vi "Logistic CDF.vi"(9 "b":dbl=1.0, 10 "a":dbl=1.0, 11 "x":dbl) -> (0 "error":i32, 3 "cdf(x)":dbl=0.2689414213699951)   [LabVIEW 2017, in "NI_Gmath.lvlib"]
doc: "Computes the continuous cumulative distribution function (CDF), or the probability that the random variate X, where X describes the selected distribution type, has a value less than or equal to <B>x</B>. You must manually select the polymorphic instance to use."
uses:
  <vilib>/gmath/NI_Gmath.lvlib
  <vilib>/gmath/statdist.llb/st_error_code.ctl
panel:
  # "Logistic CDF"
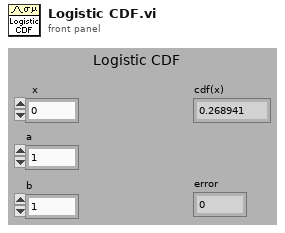
[diagram p1: front panel]
types:
  T1 = typedef "NI_Gmath.lvlib/st_error_code.ctl" = i32
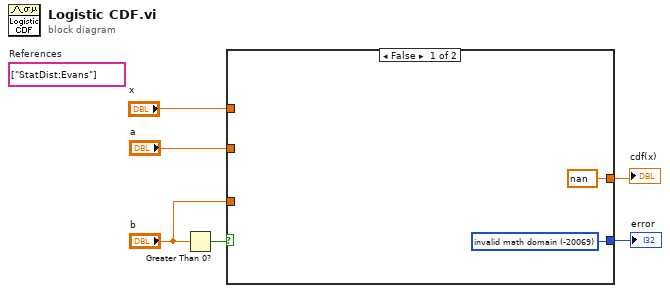
[diagram p0: block diagram]
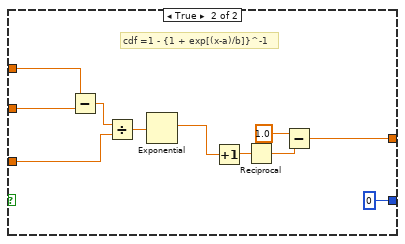
[diagram p2: hidden frame]
diagram:
  (unwired) string[] ["StatDist:Evans"]  # References
  n1 = Greater Than 0?(x="b") -> (x > 0?=w1:bool)
  n2 = case shown="False" w1 {
    tunnel: "b" -> [_ w14]
    tunnel: [w7 0 ("invalid math domain")] -> w2
    tunnel: [nan w9] -> w3
    tunnel: "x" -> [_ w18]
    tunnel: "a" -> [_ w17]
    frame False {
      w7 = T1 -20069 items=["invalid math domain"=-20069, "Fourier interpolation size m >= n"=-20070, "empty array"=-20003] ("stat interp error code")
    }
    frame True {
      # "cdf =1 - {1 + exp[(x-a)/b]}^-1"
      n3 = Subtract(x=w18, y=w17) -> (x-y=w16:dbl)
      n4 = Divide(x=w16, y=w14) -> (x/y=w15:dbl)
      n5 = Exponential(1:w15) -> (0:w13:dbl)
      n6 = Increment(x=w13) -> (x+1=w11:dbl)
      n7 = Reciprocal(x=w11) -> (1/x=w10:dbl)
      n8 = Subtract(x=1.0, y=w10) -> (x-y=w9:dbl)
    }
  }
  "cdf(x)" <- w3
  "error" <- w2
